vi "Open.vi"(8 "error in (no error)":errorcluster, 10 "Link":cluster{"IP":string, "Port":u32}, 11 "E5071C in":refnum<class "E5071C.lvclass">) -> (0 "error out":errorcluster, 2 "Link_OK":bool, 3 "E5071C out":refnum<class "E5071C.lvclass">)   [LabVIEW 2020, in "E5071C.lvlib" / "E5071C.lvclass"]
uses:
  E5071C.lvclass
  E5071C.lvclass/E5071C.ctl
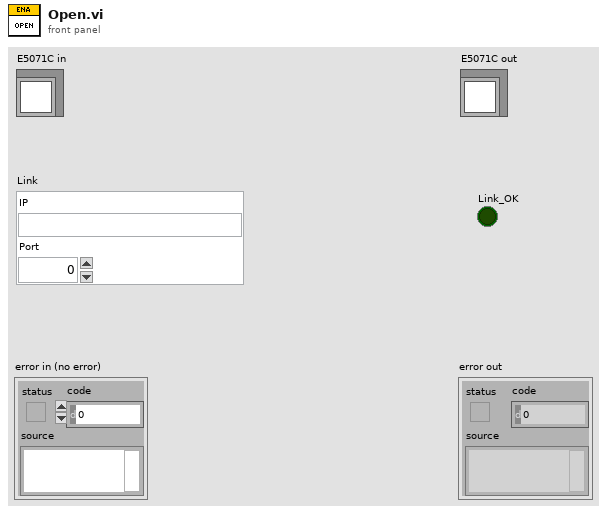
[diagram p1: front panel]
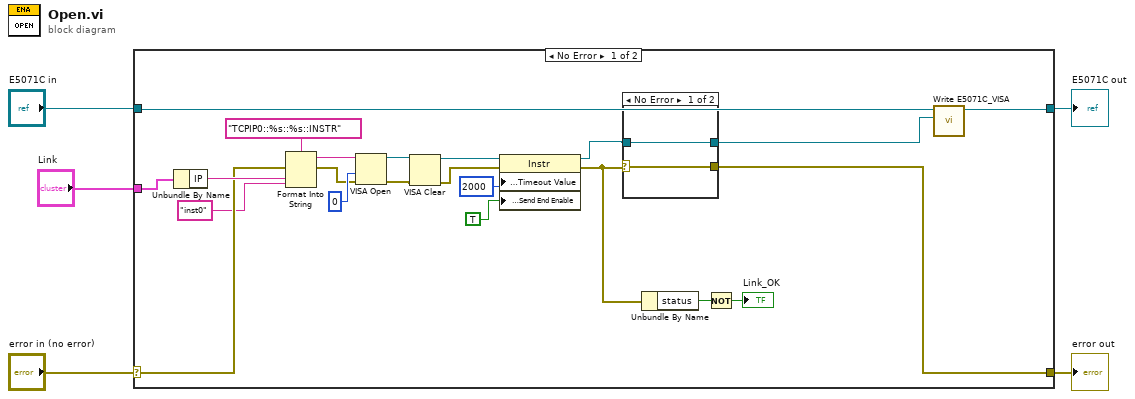
[diagram p0: block diagram]
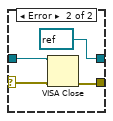
[diagram p2: hidden frame]
diagram:
  n1 = case shown="No Error" "error in (no error)" {
    selector: "error in (no error)" -> [w21 w35]
    tunnel: [w14 w35] -> w4
    tunnel: [w6 w34] -> w2
    tunnel: "E5071C in" -> [w8 w34]
    tunnel: "Link" -> [w26 _]
    frame No Error {
      n2 = Unbundle By Name(w26) -> ("IP"=w24:string)
      n3 = Format Into String(format string="TCPIP0::%s::%s::INSTR", error in=w21, w24, "inst0" ("input 2")) -> (resulting string=w23:string, error out=w22:errorcluster)  [unwired: 1 in]
      n4 = VISA Open(access mode=u32 0, error in (no error)=w22, VISA resource name=w23) -> (VISA resource name=w16:refnum<visa-resource-name>, error out=w15:errorcluster)  [unwired: 2 in]
      n5 = VISA Clear(VISA resource name=w16, error in (no error)=w15) -> (VISA resource name out=w18:refnum<visa-resource-name>, error out=w17:errorcluster)
      n6 = property class="Instr"(reference=w18, error in=w17, "General Settings:Timeout Value"=u32 2000, "Message Based Settings:Send End Enable"=TRUE) -> (reference out=w13:refnum<visa-resource-name>, error out=w12:errorcluster)
      n7 = case shown="No Error" w12 {
        selector: w12 -> [w28 w32]
        tunnel: w13 -> [w29 w30]
        tunnel: [w29 refnum<visa-resource-name> refnum ("VISA resource name out")] -> w7
        tunnel: [w28 w31] -> w14
        frame No Error {
        }
        frame Error {
          n8 = VISA Close(VISA resource name=w30, error in (no error)=w32) -> (error out=w31:errorcluster)
        }
      }
      n9 = Unbundle By Name(w12) -> ("status"=w11:bool)
      n10 = Not(x=w11) -> (.not. x?=→"Link_OK":bool)
      n11 = call "Write E5071C_VISA.vi"("E5071C_VISA"=w7, "E5071C in"=w8) -> ("E5071C out"=w6:refnum<class "E5071C.lvclass">)  [unwired: 8 in, 1 out]
    }
    frame Error {
    }
  }
  "error out" <- w4
  "E5071C out" <- w2
